vi "Shutdown.vi"(8 "error in (no error)":errorcluster, 11 "Handle in":refnum<class "Handle.lvclass">) -> (0 "error out":errorcluster, 3 "Handle out":refnum<class "Handle.lvclass">)   [LabVIEW 2021, in "Autocomplete Textbox.lvlib" / "Handle.lvclass"]
uses:
  Handle.lvclass
  ToMain UE.ctl
  ToMain UE action.ctl
  Handle.lvclass/Handle.ctl
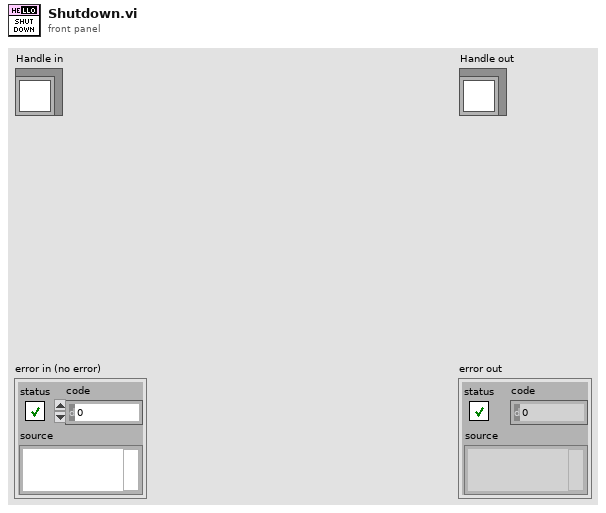
[diagram p1: front panel]
types:
  T1 = typedef "Autocomplete Textbox.lvlib/Handle.lvclass/ToMain UE.ctl" = cluster{"Type":T2, "data":variant}
  T2 = typedef "Autocomplete Textbox.lvlib/Handle.lvclass/ToMain UE action.ctl" = enum16{"New List", "Shutdown", "New Value", "Mouse Down (signal)"}
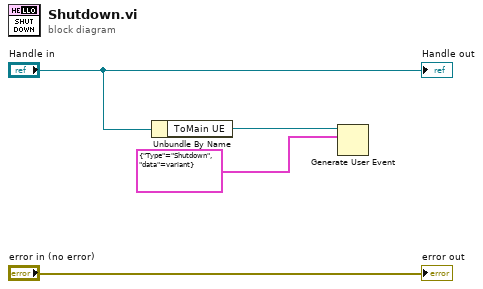
[diagram p0: block diagram]
diagram:
  n1 = Unbundle By Name("Handle in") -> ("ToMain UE"=w3:refnum<user-event>)
  n2 = Generate User Event(user event=w3, event data cluster=T1 {"Type"=enum."Shutdown", "data"=variant} ("event data")) -> ()  [unwired: 2 in, 2 out]
  "error out" <- "error in (no error)"
  "Handle out" <- "Handle in"
